vi "Write Multiple Coils.vi"(7 "unit ID":u8, 8 "error in":errorcluster, 9 "coils to write":bool[](array[boolean]), 10 "starting address":u16, 11 "Modbus master in":refnum<class "Modbus Master.lvclass">) -> (0 "error out":errorcluster, 3 "Modbus master out":refnum<class "Modbus Master.lvclass">)   [LabVIEW 2013, in "Modbus Library - Advance.lvlib" / "Modbus Master.lvclass"]
doc: "Writes <B>coils to write</B> starting at <B>starting address</B> to the device coils."
uses:
  Modbus Master.lvclass
  Modbus Master.lvclass/Modbus Master.ctl
  Modbus API.lvclass/Modbus API.ctl
  Transmission Data Unit/Transmission Data Unit.lvclass/Transmission Data Unit.ctl
  Transmission Data Unit/Transmission Data Unit.lvclass
  Master Function Definition/Master Function Definition.lvclass
  Modbus API.lvclass
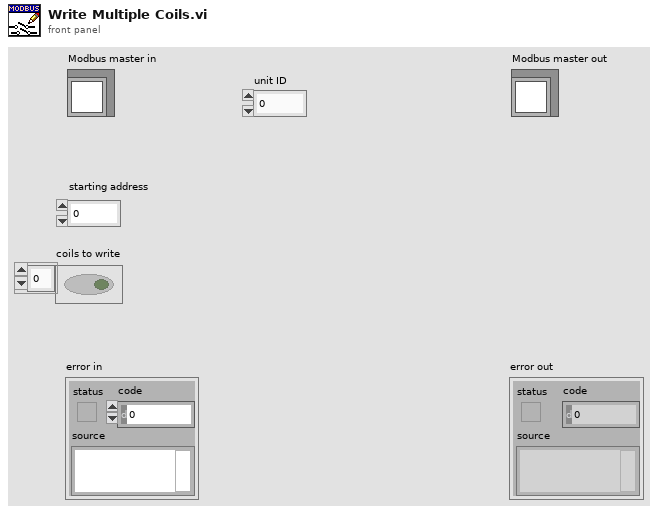
[diagram p1: front panel]
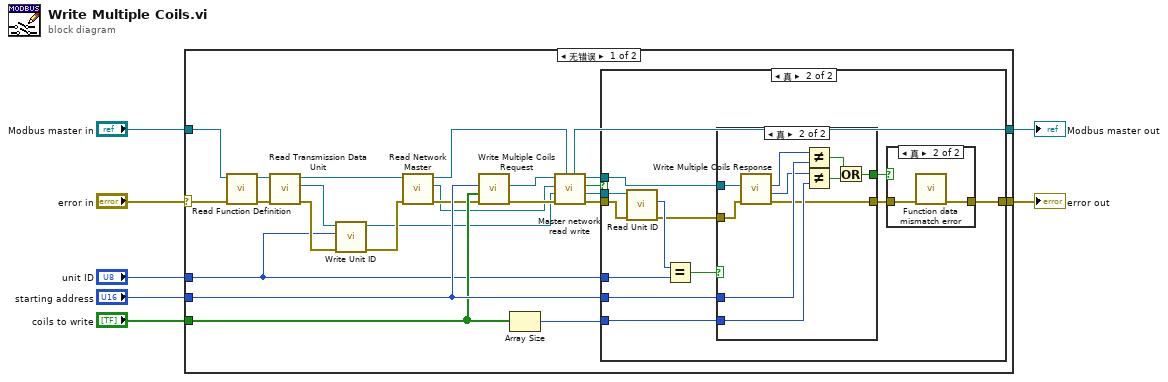
[diagram p0: block diagram]
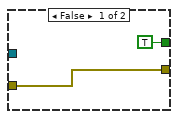
[diagram p3: hidden frame]
diagram:
  n1 = case shown="无错误" "error in" {
    selector: "error in" -> [w19 w61]
    tunnel: "Modbus master in" -> [w15 w60]
    tunnel: [w30 w61] -> w6
    tunnel: [w23 w60] -> w7
    tunnel: "starting address" -> [w29 _]
    tunnel: "coils to write" -> [w28 _]
    tunnel: "unit ID" -> [w8 _]
    frame No Error {
      n2 = call "Read Function Definition.vi"("error in"=w19, "Modbus master in"=w15) -> ("error out"=w20:errorcluster, "Modbus master out"=w21:refnum<class "Modbus Master.lvclass">)  [unwired: 7 in, 1 out]
      n3 = call "Read Transmission Data Unit.vi"("error in"=w20, "Modbus instance in"=w21) -> ("error out"=w12:errorcluster, "transmission data unit"=w13:refnum<class "Transmission Data Unit.lvclass">, "Modbus instance out"=w22:refnum<class "Modbus Master.lvclass">)  [unwired: 7 in]
      n4 = call "Write Unit ID.vi"("error in"=w12, "unit ID"=w8, "transmission data unit in"=w13) -> ("error out"=w11:errorcluster, "transmission data unit out"=w10:refnum<class "Transmission Data Unit.lvclass">)  [unwired: 7 in]
      n5 = call "Read Network Master.vi"("error in"=w11, "Modbus master in"=w22) -> ("error out"=w18:errorcluster, "network master"=w16:refnum<class "Network Master.lvclass">, "Modbus master out"=w17:refnum<class "Modbus Master.lvclass">)  [unwired: 7 in]
      n6 = call "Write Multiple Coils Request.vi"("error in"=w18, "Coils To Write"=w28, "Starting Address"=w29) -> ("error out"=w31:errorcluster, "modbus data unit out"=w24:refnum<class "Modbus Data Unit.lvclass">)  [unwired: 7 in]
      n7 = Array Size(array=w28) -> (size(s)=w27:i32)
      n8 = call "Master network read write.vi"("Modbus master in"=w17, "error in"=w31, "transmission data unit in"=w10, "network master in"=w16, "Modbus data unit in"=w24) -> ("error out"=w26:errorcluster, "transmission data unit out"=w9:refnum<class "Transmission Data Unit.lvclass">, "PDU Valid?"=w14:bool, "Modbus data unit out"=w25:refnum<class "Modbus Data Unit.lvclass">, "Modbus master out"=w23:refnum<class "Modbus Master.lvclass">)  [unwired: 2 in]
      n9 = case shown="真" w14 {
        tunnel: [w32 w43] -> w30
        tunnel: w29 -> [_ w42]
        tunnel: w27 -> [_ w41]
        tunnel: w26 -> [w32 w37]
        tunnel: w25 -> [_ w40]
        tunnel: w9 -> [_ w38]
        tunnel: w8 -> [_ w35]
        frame False {
        }
        frame True {
          n10 = call "Read Unit ID.vi"("error in"=w37, "transmission data unit in"=w38) -> ("error out"=w34:errorcluster, "unit ID"=w36:u8)  [unwired: 7 in, 1 out]
          n11 = Equal?(x=w36, y=w35) -> (x = y?=w33:bool)
          n12 = case shown="真" w33 {
            tunnel: [TRUE w56] -> w44
            tunnel: w42 -> [_ w52]
            tunnel: w41 -> [_ w50]
            tunnel: w40 -> [_ w49]
            tunnel: [w46 w48] -> w39
            tunnel: w34 -> [w46 w47]
            frame False {
            }
            frame True {
              n13 = call "Write Multiple Coils Response.vi"("error in"=w47, "modbus data unit in"=w49) -> ("error out"=w48:errorcluster, "Number of Coils"=w51:u16, "Start Address"=w53:u16)  [unwired: 7 in]
              n14 = Not Equal?(x=w53, y=w52) -> (x != y?=w55:bool)
              n15 = Not Equal?(x=w51, y=w50) -> (x != y?=w54:bool)
              n16 = Or(x=w55, y=w54) -> (x .or. y?=w56:bool)
            }
          }
          n17 = case shown="真" w44 {
            tunnel: [w57 w58] -> w43
            tunnel: w39 -> [w57 w59]
            frame False {
            }
            frame True {
              n18 = call "Function data mismatch error.vi"("error in (no error)"=w59) -> ("error out"=w58:errorcluster)  [unwired: 10 in]
            }
          }
        }
      }
    }
    frame Error {
    }
  }
  "error out" <- w6
  "Modbus master out" <- w7
